vi "Required Buffer Size (Transfer).vi"(8 "error in (no error)":errorcluster, 11 "Transfer Configuration in":T1 {"channels"."string offset" format="%d bytes"}) -> (0 "error out":errorcluster, 1 "engine buffer size":u64 format="%d bytes", 2 "string buffer size":u64 format="%d bytes", 3 "Transfer Configuration out":T1 {"channels"."string offset" format="%d bytes"})   [LabVIEW 2017, in "DSF Core.lvlib" / "Configuration Session.lvclass"]
uses:
  Configuration Session.lvclass
  Typedefs/DSF Engine Transfer Configuration.ctl
  Typedefs/DSF Byte Order.ctl
  Typedefs/DSF Settings Info.ctl
  Typedefs/DSF Engine Channel Configuration.ctl
  Typedefs/DSF Data Type.ctl
  Framework/Framework.lvclass
  DSF Core.lvlib
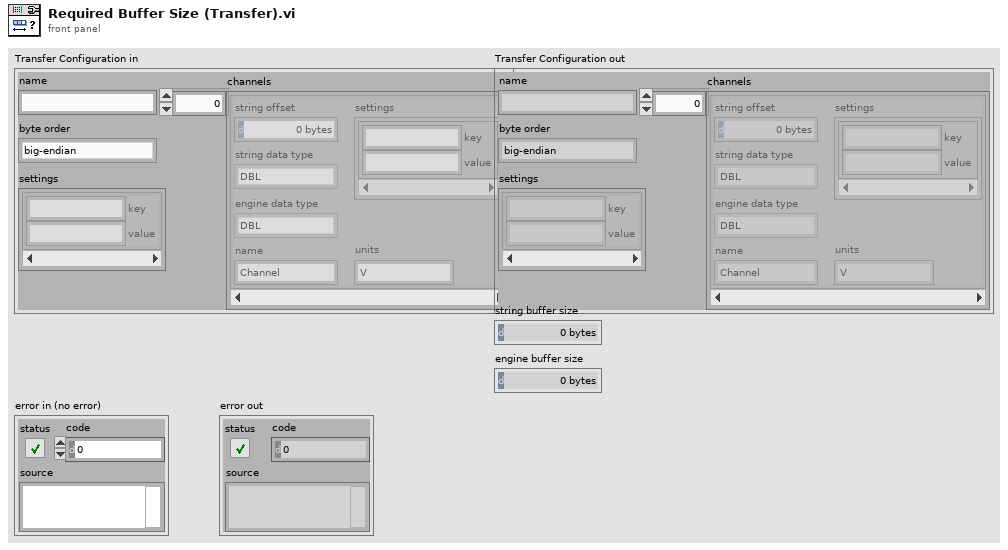
[diagram p1: front panel]
types:
  T1 = typedef "DSF Core.lvlib/DSF Engine Transfer Configuration.ctl" = cluster{"name":string, "byte order":T2, "settings":T3, "channels":T4[]}
  T2 = typedef "DSF Core.lvlib/DSF Byte Order.ctl" = enum8{"big-endian", "little-endian"}
  T3 = typedef "DSF Core.lvlib/DSF Settings Info.ctl" = cluster{"key":string, "value":string}[]
  T4 = typedef "DSF Core.lvlib/DSF Engine Channel Configuration.ctl" = cluster{"string offset":u64, "string data type":T5, "engine data type":T5, "name":string, "settings":T3, "units":string}
  T5 = typedef "DSF Core.lvlib/DSF Data Type.ctl" = enum8{"Bool", "SGL", "DBL", "I8", "I16", "I32", "I64", "U8", "U16", "U32", "U64"}
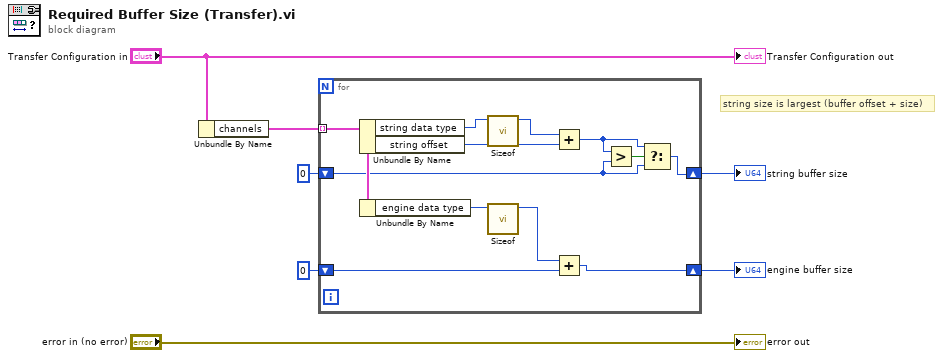
[diagram p0: block diagram]
diagram:
  # "string size is largest (buffer offset + size)"
  n1 = Unbundle By Name("Transfer Configuration in") -> ("channels"=w5:T4[])
  n2 = for {
    tunnel: w5 -> [w15] mode=indexing
    shift-right: [w17] -> w4
    shift-left: u64 0 -> [w14]
    shift-right: [w8] -> w3
    shift-left: u64 0 -> [w9]
    n3 = Unbundle By Name(w15) -> ("string data type"=w13:T5, "string offset"=w19:u64)
    n4 = Unbundle By Name(w15) -> ("engine data type"=w11:T5)
    n5 = call "Sizeof.vi"("data type"=w13) -> ("size in bytes"=w12:u64)  [unwired: 9 in, 1 out]
    n6 = call "Sizeof.vi"("data type"=w11) -> ("size in bytes"=w10:u64)  [unwired: 9 in, 1 out]
    n7 = Add(x=w12, y=w19) -> (x+y=w16:u64)
    n8 = Add(x=w10, y=w9) -> (x+y=w8:u64)
    n9 = Greater?(x=w16, y=w14) -> (0:w18:bool)
    n10 = Select(t=w16, s=w18, f=w14) -> (s? t:f=w17:u64)
  }
  "string buffer size" <- w4
  "engine buffer size" <- w3
  "Transfer Configuration out" <- "Transfer Configuration in"
  "error out" <- "error in (no error)"
